vi "Test_RegisterForWrongType_Listbox_Error.vi"(8 "error in (no error)":errorcluster, 11 "TestActorEvents In":refnum<class "TestActorEvents.lvclass">) -> (0 "error out":errorcluster, 3 "TestActorEvents Out":refnum<class "TestActorEvents.lvclass">)   [LabVIEW 2020, in "TestActorEvents.lvclass"]
uses:
  TestActorEvents.lvclass
  TestActorEvents.lvclass/TestActorEvents.ctl
  Source/IViewModel/IViewModel/IViewModel.lvclass
  modules/mva-core/Source/Mediator/Mediator/Mediator.lvclass
  <vilib>/ActorFramework/Actor/Actor.lvclass
  modules/mva-core/Source/IModel/IModel/IModel.lvclass
  Doubles/LeakyViewable/LeakyViewable.lvclass
  Doubles/LeakyViewable/Leak Location.ctl
  <vilib>/ActorFramework/Stop Msg/Stop Msg.lvclass
  Doubles/ViewableListboxBadReg/ViewableListboxBadReg.lvclass
  5df05842-43c9-4abb-a475-a400104ef06a.vi
  C:/Git/mva-viewable/Test/Doubles/LeakyViewable/LeakyViewable.lvclass
  C:/Git/mva-viewable/Source/IViewable/IViewable/IViewable.lvclass
  C:/Git/mva-viewable/Source/ActorEvents/IEventAggregator/IEventAggregator.lvclass
  C:/Git/mva-viewable/modules/mva-core/Source/IObserver/IObserver/IObserver.lvclass
  C:/Program Files (x86)/National Instruments/LabVIEW 2020/vi.lib/ActorFramework/Actor/Actor.lvclass
  C:/Git/mva-viewable/Test/Doubles/ViewableListboxBadReg/ViewableListboxBadReg.lvclass
  C:/Git/mva-viewable/Source/IViewManager/IViewManager/IViewManager.lvclass
  C:/Git/mva-viewable/Source/IViewModel/IViewModel/IViewModel.lvclass
panel:
  out "Error Status":errorcluster
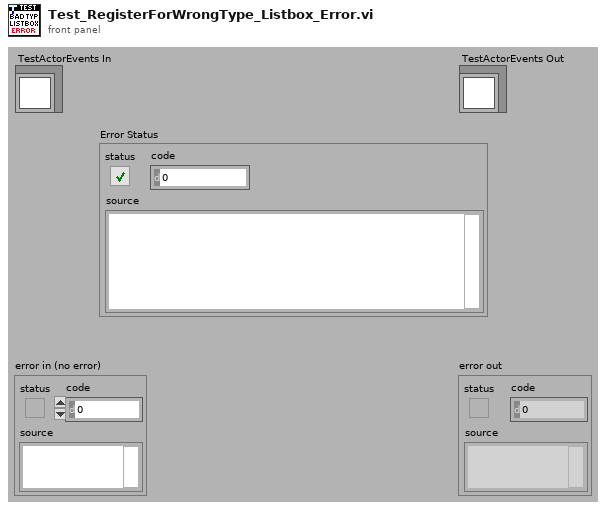
[diagram p1: front panel]
types:
  T1 = typedef "LeakyViewable.lvlib/LeakyViewable.lvclass/Leak Location.ctl" = enum16{"Pre Launch Init", "Entering Actor Core", "Actor Core", "Exiting Actor Core", "Stop Core", "Handle Error"}
  T2 = cluster{"Location":T1, "State":refnum<class "IViewable.lvclass">, "Error Status":errorcluster}
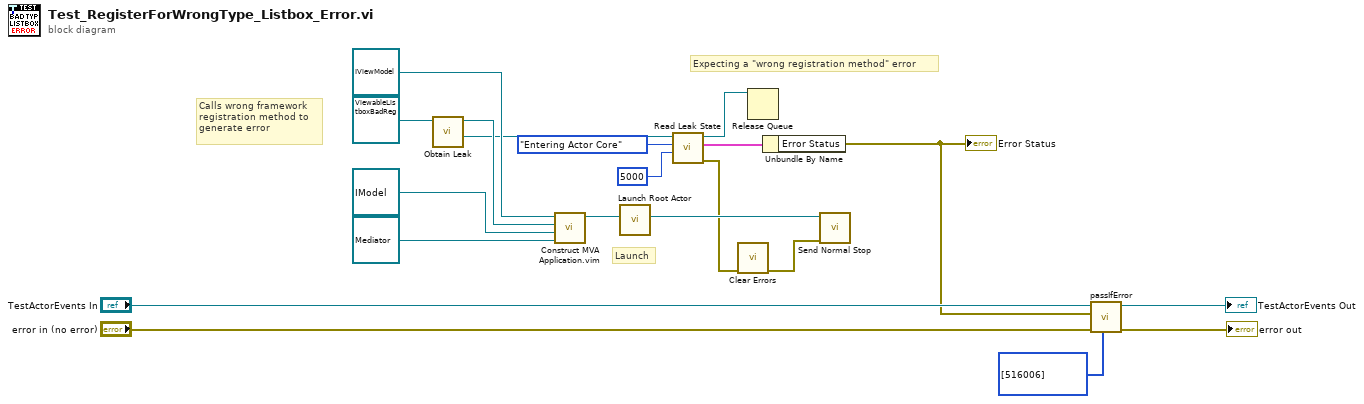
[diagram p0: block diagram]
diagram:
  # "Expecting a \"wrong registration method\" error"
  # "Calls wrong framework\nregistration method to\ngenerate error"
  # "Launch"
  n1 = call "Obtain Leak.vi"("LeakyViewable In"=refnum<class "ViewableListboxBadReg.lvclass"> refnum ("Startup View Configuration")) -> ("Viewable Leak Queue"=w9:refnum<queue>, "LeakyViewable Out"=w10:refnum<class "ViewableListboxBadReg.lvclass">)  [unwired: 9 in]
  n2 = call "Construct MVA Application.vim"("Mediator Type"=refnum<class "Mediator.lvclass"> refnum ("Mediator"), "Model Type"=refnum<class "IModel.lvclass"> refnum ("Model"), "Startup View Configuration"=w10, "IViewModel In"=refnum<class "IViewModel.lvclass"> refnum) -> ("IViewModel Out"=w12:refnum<class "IViewModel.lvclass">)  [unwired: 7 in]
  n3 = call <vilib>:"Launch Root Actor.vi"("Actor"=w12) -> ("Actor's Enqueuer"=w4:refnum<class "Message Enqueuer.lvclass">)  [unwired: 9 in, 1 out]
  n4 = call "Read Leak State.vi"("timeout in ms (-1)"=5000, "Leak Location"=Leak_Location."Entering Actor Core", "Viewable Leak Queue In"=w9) -> ("error out"=w3:errorcluster, "State Snapshot"=w6:T2, "Viewable Leak Queue"=w1:refnum<queue>)  [unwired: 5 in, 1 out]
  n5 = call <vilib>:"Clear Errors.vi"("error in (no error)"=w3) -> ("error out"=w2:errorcluster)  [unwired: 5 in, 1 out]
  n6 = Release Queue(queue=w1) -> ()  [unwired: 2 in, 3 out]
  n7 = Unbundle By Name(w6) -> ("Error Status"=w5:errorcluster)
  "Error Status" <- w5
  n8 = call <vilib>:"Send Normal Stop.vi"("error in (no error)"=w2, "Message Enqueuer"=w4) -> ()  [unwired: 9 in, 1 out]
  n9 = call-dynamic "passIfError.vi"("passing error codes (default = any error code)"=i32[] [516006], "error in (no error)"="error in (no error)", "error"=w5, "TestCase in"="TestActorEvents In") -> ("error out"=→"error out":errorcluster, "TestCase out"=→"TestActorEvents Out":refnum<class "TestActorEvents.lvclass">)  [unwired: 6 in]
